vi "ISEproject1.vi"() -> ()   [LabVIEW 2011]
uses:
  <vilib>/Analysis/NI_AALBase.lvlib
panel:
  out "Standard Deviation \nof NO3 ISE1":dbl format="%0.3f"
  out "Mean of NO3 ISE1 (V)":dbl format="%0.3f"
  out "Standard Deviation\nof PH ISE 2":dbl format="%0.3f"
  out "Standard Deviation\nof PH ISE 1":dbl format="%0.3f"
  out "Mean of PH ISE 2 (V)":dbl format="%0.3f"
  out "Mean of PH ISE 1 (V)":dbl format="%0.3f"
  out "Elapsed Time (sec)":u32
  out "Time Response Analysis of ISE":dynamicdata(graph)
  in  "stop (F)":bool
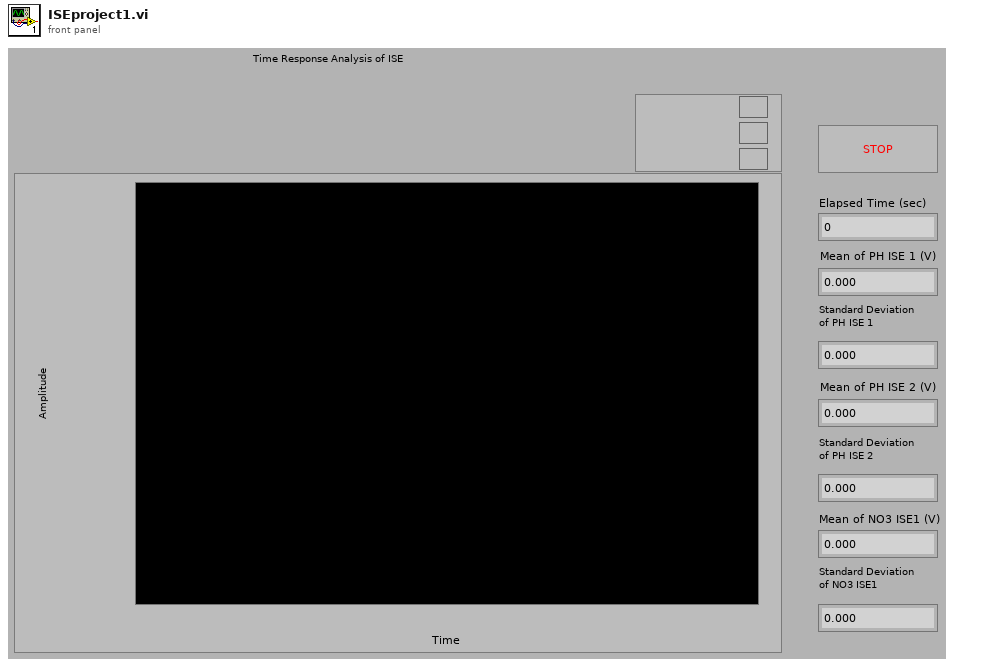
[diagram p1: front panel]
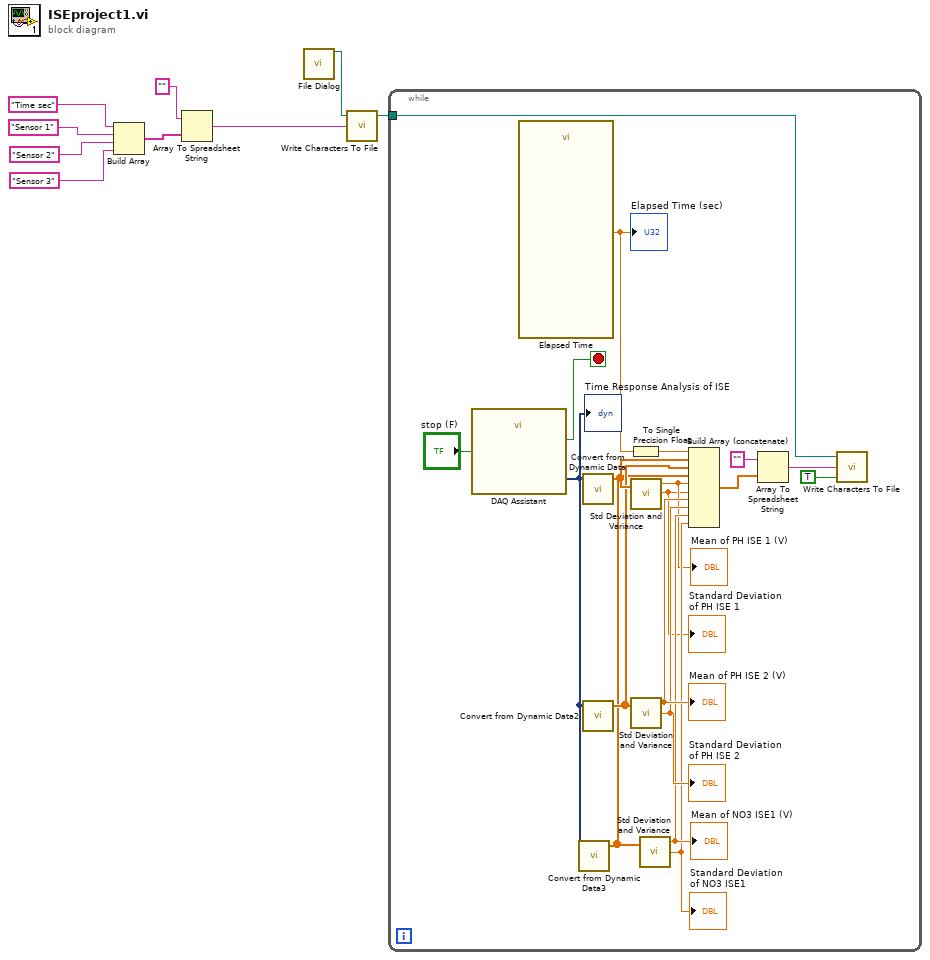
[diagram p0: block diagram]
diagram:
  n1 = Build Array "Build Array"("Time sec" ("element"), "Sensor 1" ("element"), "Sensor 2" ("element"), "Sensor 3" ("element")) -> (w4:string[])
  n2 = Array To Spreadsheet String(array=w4, 3:"" ("format string")) -> (spreadsheet string=w8:string)  [unwired: 1 out]
  n3 = call "File Dialog"() -> ("selected path"=w2:path)  [unwired: 7 in, 8 out]
  n4 = call <vilib>:"Write Characters To File.vi"("character string"=w8, "file path (dialog if empty)"=w2) -> ("new file path (Not A Path if cancelled)"=w3:path)  [unwired: 1 in, 2 out]
  n5 = while {
    tunnel: w3 -> [w26]
    stop <- w27 stop-if-true
    n6 = call "DAQ Assistant"("stop (F)"="stop (F)") -> ("data"=w17:dynamicdata, "stopped"=w27:bool)  [unwired: 4 in, 13 out]
    "Time Response Analysis of ISE" <- w17
    n7 = call "Elapsed Time"() -> ("Elapsed Time (s)"=w24:dbl)  [unwired: 5 in, 14 out]
    "Elapsed Time (sec)" <- w24
    n8 = call "Convert from Dynamic Data3"("Dynamic Data Type"=w17) -> ("Array"=w16:dbl[])  [unwired: 3 in]
    n9 = call "Convert from Dynamic Data"("Dynamic Data Type"=w17) -> ("Array"=w23:dbl[])  [unwired: 1 in, 2 out]
    n10 = call "Convert from Dynamic Data2"("Dynamic Data Type"=w17) -> ("Array"=w22:dbl[])  [unwired: 1 in, 2 out]
    n11 = To Single Precision Float(number=w24) -> (single precision float=w25:sgl)
    n12 = call <vilib>:"Std Deviation and Variance.vi"("X"=w23) -> ("mean"=w11:dbl, "standard deviation"=w10:dbl)  [unwired: 1 in, 1 out]
    "Mean of PH ISE 1 (V)" <- w11
    "Standard Deviation\nof PH ISE 1" <- w10
    n13 = call <vilib>:"Std Deviation and Variance.vi"("X"=w22) -> ("mean"=w15:dbl, "standard deviation"=w14:dbl)  [unwired: 1 in, 1 out]
    "Mean of PH ISE 2 (V)" <- w15
    "Standard Deviation\nof PH ISE 2" <- w14
    n14 = call <vilib>:"Std Deviation and Variance.vi"("X"=w16) -> ("mean"=w13:dbl, "standard deviation"=w12:dbl)  [unwired: 1 in, 1 out]
    "Mean of NO3 ISE1 (V)" <- w13
    "Standard Deviation \nof NO3 ISE1" <- w12
    n15 = Build Array (concatenate)(w25, w23, w22, w16, w11, w10, w15, w14, w13, w12) -> (w18:dbl[])
    n16 = Array To Spreadsheet String(array=w18, 3:"" ("format string")) -> (spreadsheet string=w21:string)  [unwired: 1 out]
    n17 = call <vilib>:"Write Characters To File.vi"("append to file? (new file:F)"=TRUE, "character string"=w21, "file path (dialog if empty)"=w26) -> ()  [unwired: 3 out]
  }
